vi "Name Value Metadata Start.vi"(0 "Metadata Save Path":path, 7 "Preload Metadata":path, 11 "Error In":errorcluster) -> (15 "Error Out":errorcluster)   [LabVIEW 2020]
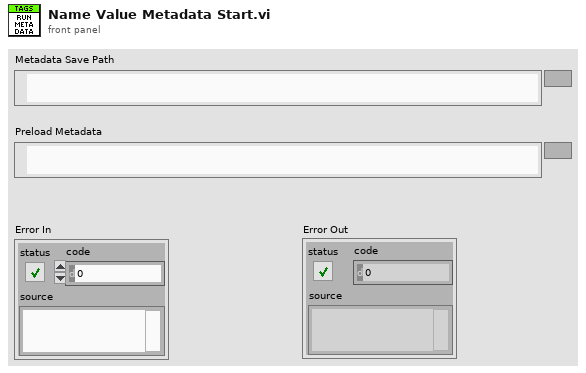
[diagram p1: front panel]
types:
  T1 = enum32{"Invalid", "Standard", "Closed", "Hidden", "Minimized", "Maximized"}
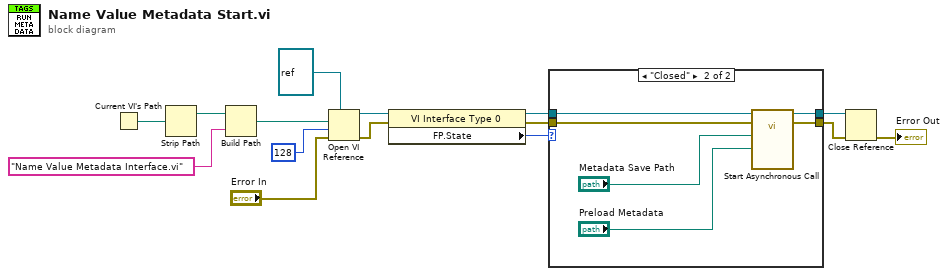
[diagram p0: block diagram]
diagram:
  n1 = Current VI's Path() -> (path=w15:path)
  n2 = Strip Path(path=w15) -> (stripped path=w14:path)  [unwired: 1 out]
  n3 = Build Path(base path=w14, name or relative path="Name Value Metadata Interface.vi") -> (appended path=w11:path)
  n4 = Open VI Reference(type specifier VI Refnum (for type only)=refnum<vi> refnum, vi path=w11, options=128, error in (no error)="Error In") -> (vi reference=w9:refnum<vi>, error out=w8:errorcluster)  [unwired: 2 in]
  n5 = property class="VI Interface Type 0"(reference=w9, error in=w8) -> (reference out=w6:refnum<vi>, error out=w5:errorcluster, "FP.State"=w7:T1)
  n6 = case shown="\"Closed\"" w7 {
    tunnel: [w17 w19] -> w3
    tunnel: w6 -> [w16 w21]
    tunnel: w5 -> [w17 w20]
    tunnel: [w16 w18] -> w4
    frame Default {
    }
    frame "Closed" {
      n7 = call-by-ref "Start Asynchronous Call"(reference=w21, error in=w20, "Save Path"="Metadata Save Path", "Input Tags Path"="Preload Metadata") -> (reference out=w18:refnum<vi>, error out=w19:errorcluster)  [unwired: 14 in]
    }
  }
  n8 = Close Reference(reference=w4, error in (no error)=w3) -> (error out=→"Error Out":errorcluster)
